vi "run_repeatingMembraneTest_pharmabot.vi"(6 "ExpPhase":string, 8 "error in":errorcluster, 9 "data in":T2={"daq_ao 1"="Dev1/ao0", "daq_ai 1"="Dev1/ai0", "experiment day folder"=path "D:/DATA/8-27-15 save func testing/test.lvm", "Multiclamp init error"=0, "Multiclamp Handle Out"=0, "sampling rate (Hz)"=10000, "trial name"=""}, 10 "misc common.stop memtest":refnum<vi>, 11 "controls array in":refnum<vi>[](array[refnum])) -> (0 "error out":errorcluster, 1 "data out":T2={"daq_ao 1"="Dev1/ao0", "daq_ai 1"="Dev1/ai0", "experiment day folder"=path "D:/DATA/8-27-15 save func testing/test.lvm", "Multiclamp init error"=0, "Multiclamp Handle Out"=0, "sampling rate (Hz)"=10000, "trial name"=""}, 2 "Cell Good?":bool, 3 "control array out":refnum<vi>[](array[refnum]), 4 "cell stats":T1 {"STD" format="%010.2f"; "Variance" format="%010.2f"; "Rt (MOhms)" format="%010.2f"; "tau (ms)" format="%08.2g"; "Cm (pF)" format="%08.2f"; "Ra (MOhms)" format="%010.2f"; "Rm (MOhms)" format="%010.2f"; "Ihold (pA)" format="%010.2f"})   [LabVIEW 2019]
uses:
  get_data_from_control_tfarray.vi
  get_data_from_control_double.vi
  wc_protocol_v1.003 Folder/whole_cell_protocol/Controls/cell_stats-v02.ctl
  Controls/Data.ctl
panel:
  out "repMemTest TF set":T3
  # "RUN repMemTest SET AUTO WC"
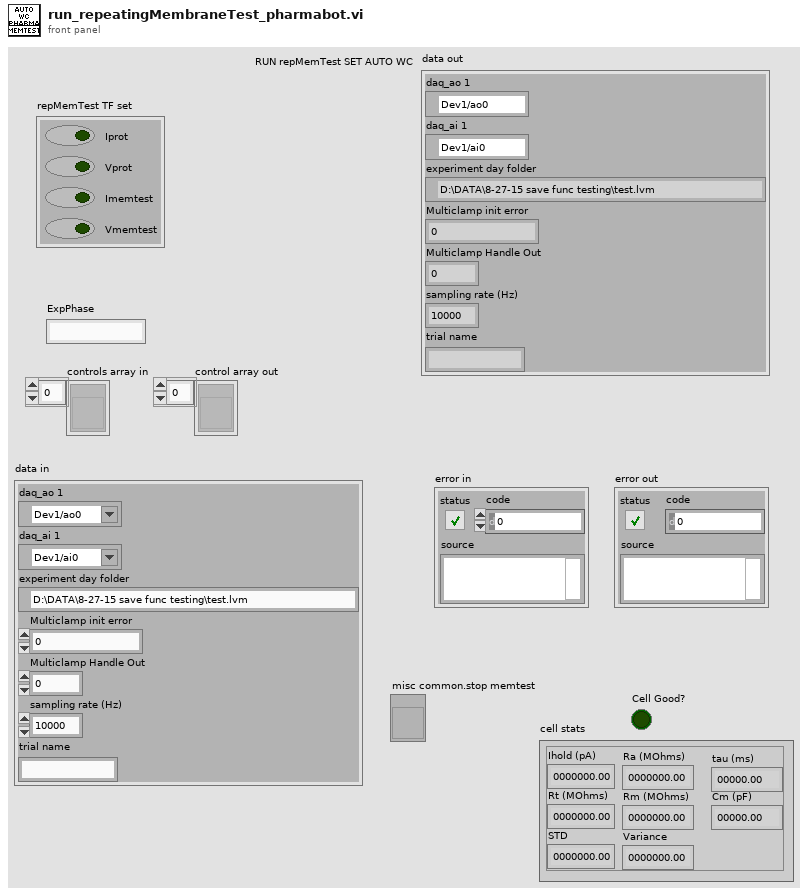
[diagram p1: front panel]
types:
  T1 = typedef "cell_stats-v02.ctl" = cluster{"Ihold (pA)":dbl, "Rm (MOhms)":dbl, "Ra (MOhms)":dbl, "Cm (pF)":dbl, "tau (ms)":dbl, "Rt (MOhms)":dbl, "Variance":dbl, "STD":dbl}
  T2 = typedef "Data.ctl" = cluster{"daq_ao 1":tag, "daq_ai 1":tag, "experiment day folder":path, "Multiclamp init error":i32, "Multiclamp Handle Out":u32, "sampling rate (Hz)":i32, "trial name":string}
  T3 = cluster{" Iprot":bool, " Vprot":bool, " Imemtest":bool, " Vmemtest":bool}
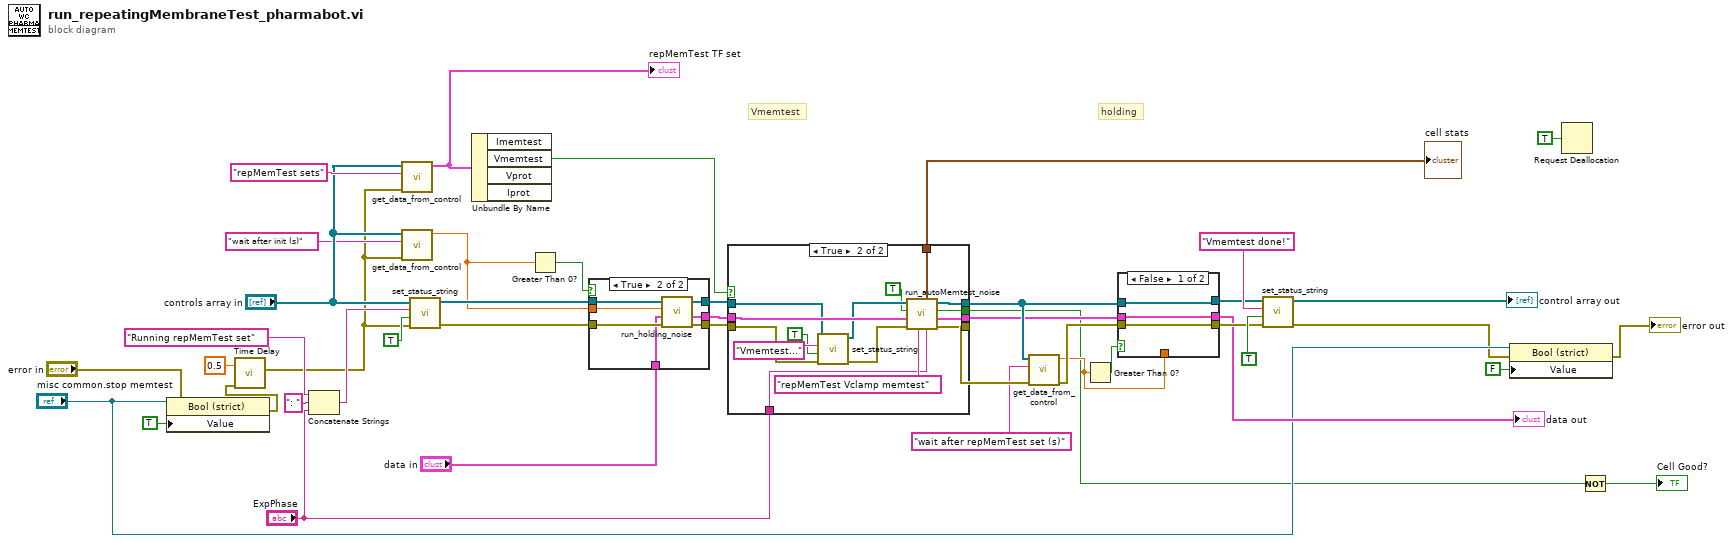
[diagram p0: block diagram]
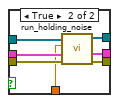
[diagram p2: hidden frame]
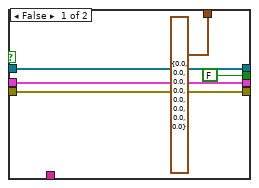
[diagram p4: hidden frame]
diagram:
  # "Vmemtest"
  # "holding"
  n1 = property class="Bool (strict)"(reference="misc common.stop memtest", error in="error in", "Value"=TRUE) -> (error out=w5:errorcluster)  [unwired: 1 out]
  n2 = call "Time Delay"("error in (no error)"=w5, "Delay Time (s)"=0.5) -> ("error out"=w7:errorcluster)  [unwired: 9 in]
  n3 = Concatenate Strings("Running repMemTest set" ("status string in"), ": " ("string"), "ExpPhase") -> (w14:string)
  n4 = call-poly "get_data_from_control.vi"("error in"=w7, "control label"="repMemTest sets", "controls array"="controls array in") -> ("TF set out"=w44:T3)  [unwired: 7 in, 1 out]
  "repMemTest TF set" <- w44
  n5 = call-poly "get_data_from_control.vi"("error in"=w7, "control label"="wait after init (s)", "controls array"="controls array in") -> ("double out"=w21:dbl)  [unwired: 7 in, 1 out]
  n6 = call "set_status_string.vi"("error in"=w7, "new line?"=TRUE, "status string in"=w14, "controls array"="controls array in") -> ("error out"=w28:errorcluster, "controls array out"=w29:refnum<vi>[])  [unwired: 6 in]
  n7 = Unbundle By Name(w44) -> ("Vmemtest"=w36:bool)  [unwired: 3 out]
  n8 = Greater Than 0?(x=w21) -> (x > 0?=w20:bool)
  n9 = case shown="True" w20 {
    tunnel: w29 -> [w47 w54]
    tunnel: w28 -> [w46 w53]
    tunnel: [w46 w52] -> w24
    tunnel: [w47 w51] -> w22
    tunnel: "data in" -> [w45 w50]
    tunnel: [w45 w49] -> w23
    tunnel: w21 -> [_ w48]
    frame False {
    }
    frame True {
      n10 = call "run_holding_noise.vi"("error in"=w53, "data in"=w50, "holding time (s)"=w48, "controls array in"=w54) -> ("error out"=w52:errorcluster, "data out"=w49:T2, "controls array out"=w51:refnum<vi>[])  [unwired: 4 in, 1 out]
    }
  }
  n11 = case shown="True" w36 {
    tunnel: w22 -> [w59 w73]
    tunnel: w24 -> [w57 w69]
    tunnel: w23 -> [w58 w74]
    tunnel: [w59 w67] -> w41
    tunnel: [w58 w66] -> w40
    tunnel: [w57 w65] -> w39
    tunnel: "ExpPhase" -> [_ w62]
    tunnel: [FALSE ("cell quality bad") w61] -> w3
    tunnel: [T1 {"Ihold (pA)"=0.0, "Rm (MOhms)"=0.0, "Ra (MOhms)"=0.0, "Cm (pF)"=0.0, "tau (ms)"=0.0, "Rt (MOhms)"=0.0, "Variance"=0.0, "STD"=0.0} ("cell stats") w60] -> w1
    frame False {
    }
    frame True {
      n12 = call "set_status_string.vi"("error in"=w69, "new line?"=TRUE, "status string in"="Vmemtest...", "controls array"=w73) -> ("error out"=w68:errorcluster, "controls array out"=w72:refnum<vi>[])  [unwired: 6 in]
      n13 = call "run_autoMemtest_noise.vi"("ExpPhase"=w62, "control label"="repMemTest Vclamp memtest", "error in"=w68, "data in"=w74, "clamp switch (T=v, F=i)"=TRUE, "controls array"=w72) -> ("error out"=w65:errorcluster, "data out"=w66:T2, "cell quality bad"=w61:bool, "controls out"=w67:refnum<vi>[], "cell stats"=w60:T1)  [unwired: 1 in]
    }
  }
  "cell stats" <- w1
  n14 = call-poly "get_data_from_control.vi"("error in"=w39, "control label"="wait after repMemTest set (s)", "controls array"=w41) -> ("error out"=w30:errorcluster, "double out"=w18:dbl)  [unwired: 7 in]
  n15 = Greater Than 0?(x=w18) -> (x > 0?=w19:bool)
  n16 = case shown="False" w19 {
    tunnel: w40 -> [w76 w84]
    tunnel: [w77 w83] -> w35
    tunnel: [w75 w82] -> w34
    tunnel: [w76 w81] -> w33
    tunnel: w41 -> [w77 w80]
    tunnel: w30 -> [w75 w79]
    tunnel: w18 -> [_ w78]
    frame False {
    }
    frame True {
      n17 = call "run_holding_noise.vi"("error in"=w79, "data in"=w84, "holding time (s)"=w78, "controls array in"=w80) -> ("error out"=w82:errorcluster, "data out"=w81:T2, "controls array out"=w83:refnum<vi>[])  [unwired: 4 in, 1 out]
    }
  }
  "data out" <- w33
  n18 = call "set_status_string.vi"("error in"=w34, "new line?"=TRUE, "status string in"="Vmemtest done!", "controls array"=w35) -> ("error out"=w9:errorcluster, "controls array out"=→"control array out":refnum<vi>[])  [unwired: 6 in]
  n19 = property class="Bool (strict)"(reference="misc common.stop memtest", error in=w9, "Value"=FALSE) -> (error out=→"error out":errorcluster)  [unwired: 1 out]
  n20 = Request Deallocation(TRUE ("flag")) -> ()
  n21 = Not(x=w3) -> (.not. x?=→"Cell Good?":bool)
